vi "Generate write queue item.vi"(8 "error in (no error)":errorcluster, 11 "Abort MsgPack in":refnum<class "Abort MsgPack.lvclass">) -> (0 "error out":errorcluster, 2 "Write queue item":T1, 3 "Abort MsgPack out":refnum<class "Abort MsgPack.lvclass">)   [LabVIEW 2020, in "wamplv.lvlib" / "Abort MsgPack.lvclass"]
uses:
  Abort MsgPack.lvclass
  Abort MsgPack.lvclass/Abort MsgPack.ctl
  cf9281e4-cdc7-4391-bfc3-c4a2100e25ce.vi
  MessagePack/MsgPackArray/MsgPackArray.lvclass
  MessagePack/MsgPackString/MsgPackString.lvclass
  TypeDefs/WAMP Message Codes.ctl
  wamplv.lvlib
  MessagePack/MsgPackMap/MsgPackMap.lvclass
  ae190724-6c1b-4e50-853a-072fc6b7fa0a.vi
  C:/local/wamplv/MessagePack/MsgPackString/MsgPackString.lvclass
  C:/local/wamplv/MessagePack/IMessagePackObject/IMessagePackObject.lvclass
  MessagePack/MessagePackNumeric/MessagePackNumeric.lvclass
  C:/local/wamplv/MessagePack/MessagePackNumeric/MessagePackNumeric.lvclass
  C:/local/wamplv/MessagePack/IMsgPackContainer/IMsgPackContainer.lvclass
  C:/local/wamplv/MessagePack/MsgPackMap/MsgPackMap.lvclass
  TypeDefs/Transport type.ctl
  WAMP Client/Private/TypeDef/Write queue item.ctl
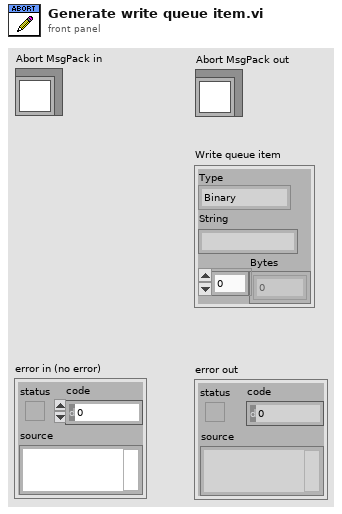
[diagram p1: front panel]
types:
  T1 = typedef "wamplv.lvlib/Write queue item.ctl" = cluster{"Type":T2, "String":string, "Bytes":u8[]}
  T2 = typedef "wamplv.lvlib/Transport type.ctl" = enum16{"Binary", "Text"}
  T3 = typedef "wamplv.lvlib/WAMP Message Codes.ctl" = enum8{"HELLO", "WELCOME", "CHALLENGE", "AUTHENTICATE", "ABORT", "GOODBYE", "ERROR", "PUBLISH", "PUBLISHED", "SUBSCRIBE", "SUBSCRIBED", "UNSUBSCRIBE", "UNSUBSCRIBED", "EVENT", "CALL", "RESULT", "REGISTER", "REGISTERED", "UNREGISTER", "UNREGISTERED", "INVOCATION", "YIELD"}
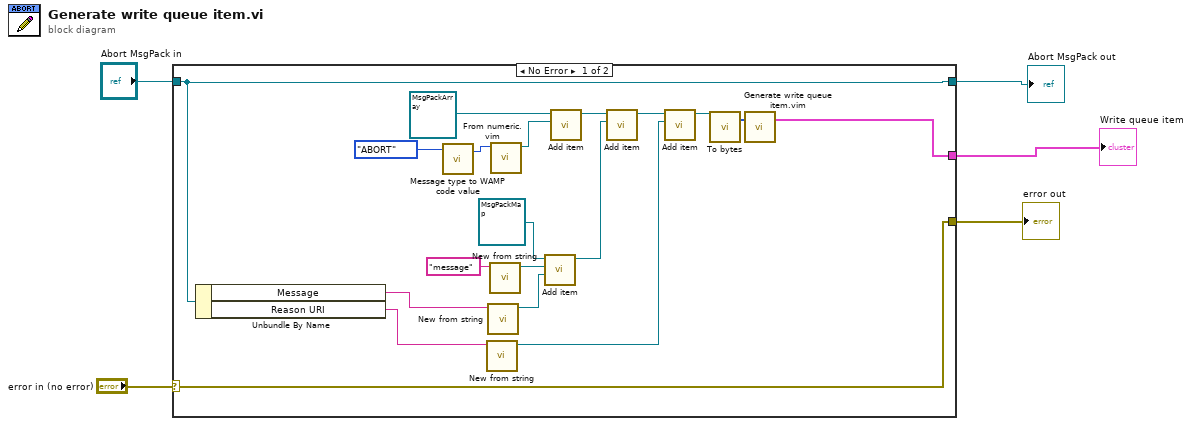
[diagram p0: block diagram]
diagram:
  n1 = case shown="No Error" "error in (no error)" {
    selector: "error in (no error)" -> [w6 w26]
    tunnel: "Abort MsgPack in" -> [w24 w25]
    tunnel: [w6 w26] -> w3
    tunnel: [w24 w25] -> w2
    tunnel: [w23 _] -> w1
    frame No Error {
      n2 = Unbundle By Name(w24) -> ("Message"=w9:string, "Reason URI"=w8:string)
      n3 = call "Message type to WAMP code value.vi"("Message Type"=WAMP_Message_Codes."ABORT" ("Message Codes")) -> ("WAMP Numeric value"=w10:u8)  [unwired: 2 in]
      n4 = call "New from string.vi"("String"=w8) -> ("output cluster"=w12:refnum<class "MsgPackString.lvclass">)  [unwired: 10 in]
      n5 = call "New from string.vi"("String"=w9) -> ("output cluster"=w19:refnum<class "MsgPackString.lvclass">)  [unwired: 10 in]
      n6 = call "New from string.vi"("String"="message") -> ("output cluster"=w18:refnum<class "MsgPackString.lvclass">)  [unwired: 10 in]
      n7 = call "From numeric.vim"("Number"=w10) -> ("MessagePackNumeric out"=w21:refnum<class "MessagePackNumeric.lvclass">)  [unwired: 10 in]
      n8 = call "Add item.vi"("Value"=w19, "Key"=w18, "MsgPackMap in"=refnum<class "MsgPackMap.lvclass"> refnum ("MessagePack.lvlib:MsgPackMap.lvclass")) -> ("MsgPackMap out"=w15:refnum<class "MsgPackMap.lvclass">)  [unwired: 8 in]
      n9 = call "Add item.vi"("wamplv.lvlib:IMessagePackObject.lvclass"=w21, "MsgPackArray in"=refnum<class "MsgPackArray.lvclass"> refnum ("MessagePack.lvlib:MsgPackArray.lvclass")) -> ("MsgPackArray out"=w16:refnum<class "MsgPackArray.lvclass">)  [unwired: 9 in]
      n10 = call "Add item.vi"("wamplv.lvlib:IMessagePackObject.lvclass"=w15, "MsgPackArray in"=w16) -> ("MsgPackArray out"=w13:refnum<class "MsgPackArray.lvclass">)  [unwired: 9 in]
      n11 = call "Add item.vi"("wamplv.lvlib:IMessagePackObject.lvclass"=w12, "MsgPackArray in"=w13) -> ("MsgPackArray out"=w14:refnum<class "MsgPackArray.lvclass">)  [unwired: 9 in]
      n12 = call-dynamic "To bytes.vi"("MsgPackArray in"=w14) -> ("Array"=w7:u8[])  [unwired: 2 in]
      n13 = call "Generate write queue item.vim"("Input"=w7) -> ("Ouput"=w23:T1)  [unwired: 2 in]
    }
    frame Error {
    }
  }
  "error out" <- w3
  "Abort MsgPack out" <- w2
  "Write queue item" <- w1
